vi "simple_tiempo_ejecución_program.vi"() -> ()   [LabVIEW 2024]
panel:
  in  "stop":bool
  out "x-y":dbl
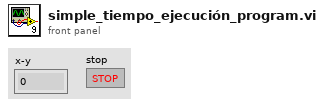
[diagram p1: front panel]
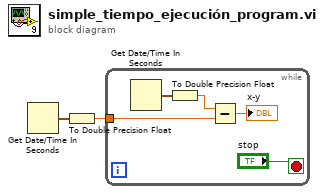
[diagram p0: block diagram]
diagram:
  n1 = Get Date/Time In Seconds() -> (seconds since 1Jan1904=w2:timestamp)
  n2 = To Double Precision Float(number=w2) -> (double precision float=w1:dbl)
  n3 = while {
    tunnel: w1 -> [w3]
    stop <- "stop" stop-if-true
    n4 = Get Date/Time In Seconds() -> (seconds since 1Jan1904=w7:timestamp)
    n5 = To Double Precision Float(number=w7) -> (double precision float=w4:dbl)
    n6 = Subtract(x=w4, y=w3) -> (x-y=→"x-y":dbl)
  }
